vi "dfd_Convert Complex Array to String.vi"(5 "indent order":i32, 6 "display in one line?":bool, 7 "format string":string="%24.16e", 11 "roots":cdb[](array[numeric]) format="%.2f") -> (3 "string":string)   [LabVIEW 2017, in "NI_DigFilter_Process.lvlib"]
uses:
  <vilib>/addons/Digital Filter Design/NI_DigFilter_Process.lvlib
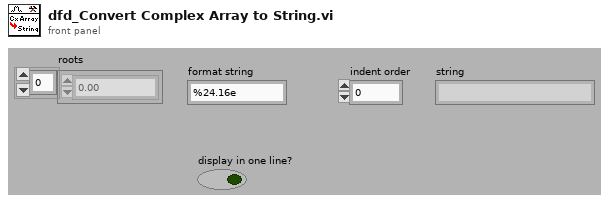
[diagram p1: front panel]
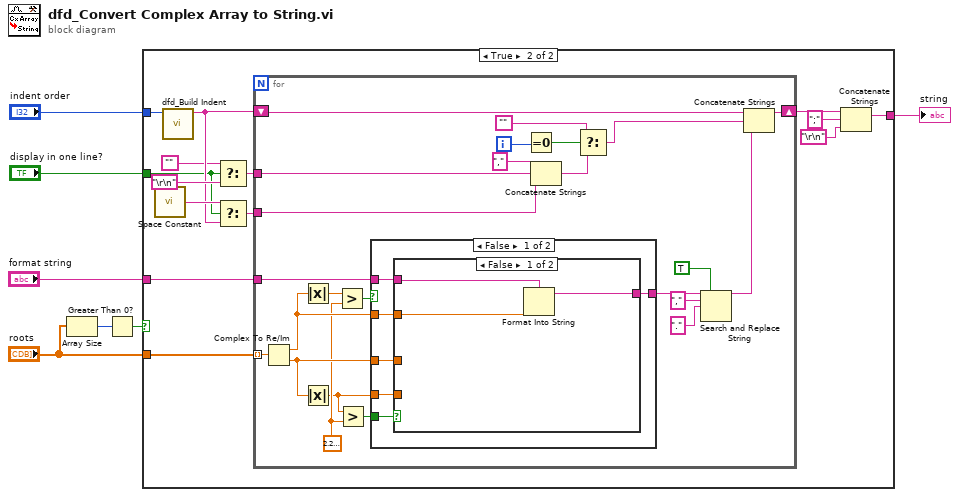
[diagram p0: block diagram]
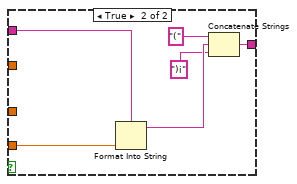
[diagram p3: hidden frame]
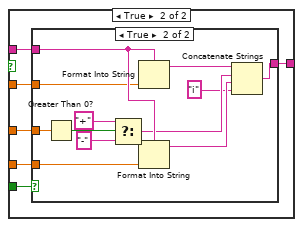
[diagram p4: hidden frame]
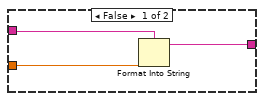
[diagram p5: hidden frame]
diagram:
  n1 = Array Size(array="roots") -> (size(s)=w2:i32)
  n2 = Greater Than 0?(x=w2) -> (x > 0?=w3:bool)
  n3 = case shown="True" w3 {
    tunnel: "roots" -> [_ w15]
    tunnel: "format string" -> [_ w21]
    tunnel: "indent order" -> [_ w17]
    tunnel: [_ w19] -> w5
    tunnel: "display in one line?" -> [_ w8]
    frame False {
    }
    frame True {
      n4 = call <vilib>:"Space Constant.vi"() -> ("String"=w14:string)
      n5 = call <vilib>:"dfd_Build Indent.vi"("indent order"=w17) -> ("tag indent"=w11:string)  [unwired: 10 out]
      n6 = Select(t="", s=w8, f="\r\n") -> (s? t:f=w12:string)
      n7 = Select(t=w14, s=w8, f=w11) -> (s? t:f=w10:string)
      n8 = for {
        tunnel: w15 -> [w37] mode=indexing
        shift-right: [w43] -> w20
        shift-left: w11 -> [w42]
        tunnel: w21 -> [w38]
        tunnel: w10 -> [w28]
        tunnel: w12 -> [w27]
        i -> [w44]
        w32 = 2.220446049250313e-16
        n9 = Complex To Re/Im(x + iy=w37) -> (x=w35:dbl, y=w36:dbl)
        n10 = Absolute Value(x=w35) -> (abs(x)=w34:dbl)
        n11 = Absolute Value(x=w36) -> (abs(x)=w30:dbl)
        n12 = Greater?(x=w34, y=w32) -> (0:w33:bool)
        n13 = Greater?(x=w30, y=w32) -> (0:w31:bool)
        n14 = case shown="False" w33 {
          tunnel: w38 -> [w51 w66]
          tunnel: w35 -> [w50 w65]
          tunnel: w30 -> [w48 w64]
          tunnel: w36 -> [w49 w63]
          tunnel: w31 -> [w47 w62]
          tunnel: [w46 w61] -> w24
          frame False {
            n15 = case shown="False" w47 {
              tunnel: w51 -> [w54 w56]
              tunnel: w50 -> [w53 _]
              tunnel: w48 -> [_ w60]
              tunnel: w49 -> [_ _]
              tunnel: [w52 w58] -> w46
              frame False {
                n16 = Format Into String(format string=w54, w53) -> (resulting string=w52:string)  [unwired: 2 in, 1 out]
              }
              frame True {
                n17 = Format Into String(format string=w56, w60) -> (resulting string=w59:string)  [unwired: 2 in, 1 out]
                n18 = Concatenate Strings("(" ("string"), w59, ")i" ("string")) -> (w58:string)
              }
            }
          }
          frame True {
            n19 = case shown="True" w62 {
              tunnel: w66 -> [w69 w81]
              tunnel: w65 -> [w68 w80]
              tunnel: w64 -> [_ w78]
              tunnel: w63 -> [_ w77]
              tunnel: [w67 w72] -> w61
              frame False {
                n20 = Format Into String(format string=w69, w68) -> (resulting string=w67:string)  [unwired: 2 in, 1 out]
              }
              frame True {
                n21 = Greater Than 0?(x=w77) -> (x > 0?=w76:bool)
                n22 = Select(t="+", s=w76, f="-") -> (s? t:f=w71:string)
                n23 = Format Into String(format string=w81, w80) -> (resulting string=w79:string)  [unwired: 2 in, 1 out]
                n24 = Format Into String(format string=w81, w78) -> (resulting string=w73:string)  [unwired: 2 in, 1 out]
                n25 = Concatenate Strings(w79, w71, w73, "i" ("string")) -> (w72:string)
              }
            }
          }
        }
        n26 = Equal To 0?(x=w44) -> (x = 0?=w45:bool)
        n27 = Concatenate Strings(",", w27, w28) -> (w39:string)
        n28 = Select(t="", s=w45, f=w39) -> (s? t:f=w41:string)
        n29 = Search and Replace String(replace all?=TRUE ("replace all? (F)"), input string=w24, search string=",", replace string="." ("replace string (\"\")")) -> (result string=w23:string)  [unwired: 1 in, 6 out]
        n30 = Concatenate Strings(w42, w41, w23) -> (w43:string)
      }
      n31 = Concatenate Strings(w20, ";" ("string"), "\r\n") -> (w19:string)
    }
  }
  "string" <- w5
